vi "Configure Internal Sweep Source.vi"(5 "Number Of Steps (1)":i32=1, 6 "Log Step (2.6922)":dbl=2.6922, 7 "Linear Step (0)":i32, 8 "error in (no error)":errorcluster, 9 "Source Axis (0: swpOut)":i32(ring) items=["swpInner", "swpOuter"], 10 "Enable Log (T: Enable)":bool=TRUE, 11 "VISA resource name":refnum<visa-resource-name>) -> (0 "error out":errorcluster, 3 "VISA resource name out":refnum<visa-resource-name>)   [LabVIEW 2014, in "Stanford Research SR1.lvlib"]
doc: "Configures the attributes of the Internal Sweep Source."
uses:
  Stanford Research SR1.lvlib
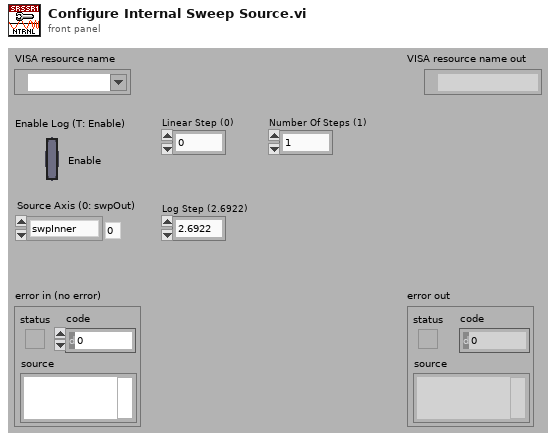
[diagram p1: front panel]
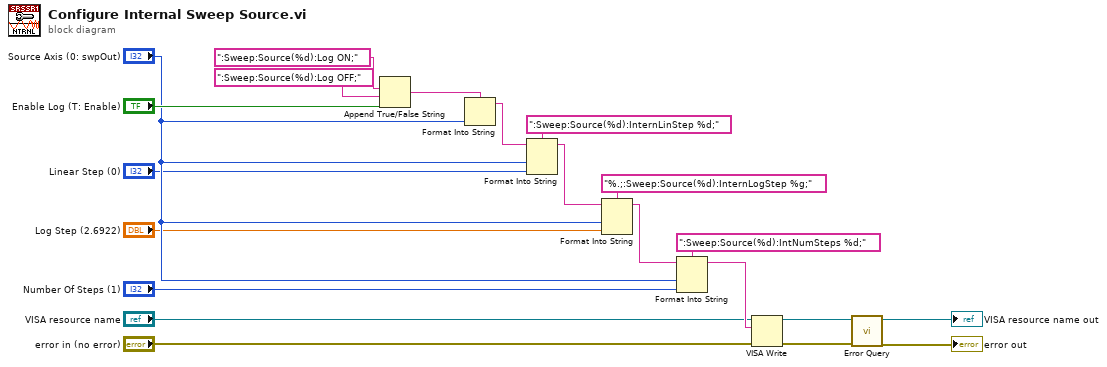
[diagram p0: block diagram]
diagram:
  n1 = Append True/False String(1:"Enable Log (T: Enable)", 2:":Sweep:Source(%d):Log OFF;", 3:":Sweep:Source(%d):Log ON;") -> (0:w6:string)  [unwired: 1 in]
  n2 = Format Into String(format string=w6, "Source Axis (0: swpOut)") -> (resulting string=w4:string)  [unwired: 2 in, 1 out]
  n3 = Format Into String(format string=":Sweep:Source(%d):InternLinStep %d;", initial string=w4, "Source Axis (0: swpOut)", "Linear Step (0)") -> (resulting string=w17:string)  [unwired: 1 in, 1 out]
  n4 = Format Into String(format string="%.;:Sweep:Source(%d):InternLogStep %g;", initial string=w17, "Source Axis (0: swpOut)", "Log Step (2.6922)") -> (resulting string=w15:string)  [unwired: 1 in, 1 out]
  n5 = Format Into String(format string=":Sweep:Source(%d):IntNumSteps %d;", initial string=w15, "Source Axis (0: swpOut)", "Number Of Steps (1)") -> (resulting string=w13:string)  [unwired: 1 in, 1 out]
  n6 = VISA Write(VISA resource name="VISA resource name", write buffer=w13, error in (no error)="error in (no error)") -> (VISA resource name out=w10:refnum<visa-resource-name>, error out=w9:errorcluster)  [unwired: 1 out]
  n7 = call "Error Query.vi"("error in (no error)"=w9, "VISA resource name"=w10) -> ("error out"=→"error out":errorcluster, "VISA resource name out"=→"VISA resource name out":refnum<visa-resource-name>)  [unwired: 6 in, 2 out]
